vi "GetRow.vi"(0 "reference in":refnum<class "DataGridView.lvclass">, 5 "index":i32, 11 "error in (no error)":errorcluster) -> (4 "reference out":refnum<class "DataGridView.lvclass">, 6 "Array":refnum<k24>[](array[refnum]), 15 "error out":errorcluster)   [LabVIEW 2018, in "DataGridView.lvclass"]
doc: "Gets the row by index"
uses:
  DataGridView.lvclass
  System.Windows.Forms
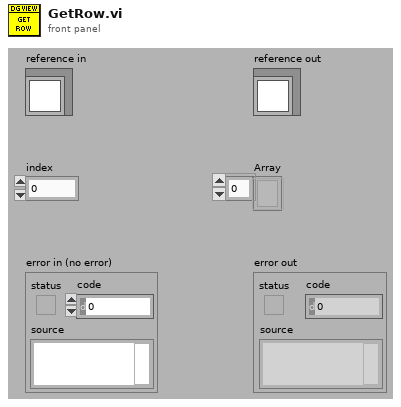
[diagram p1: front panel]
types:
  T1 = typedef "DataGridView.lvclass/ObjectAttributes.ctl" = cluster{"DataGridView":refnum<k24>, "SelectionChangedEvent":refnum<user-event>, "SelectionChanged callback ref":refnum<k27>, "LastSelectedRowIndex":i32}
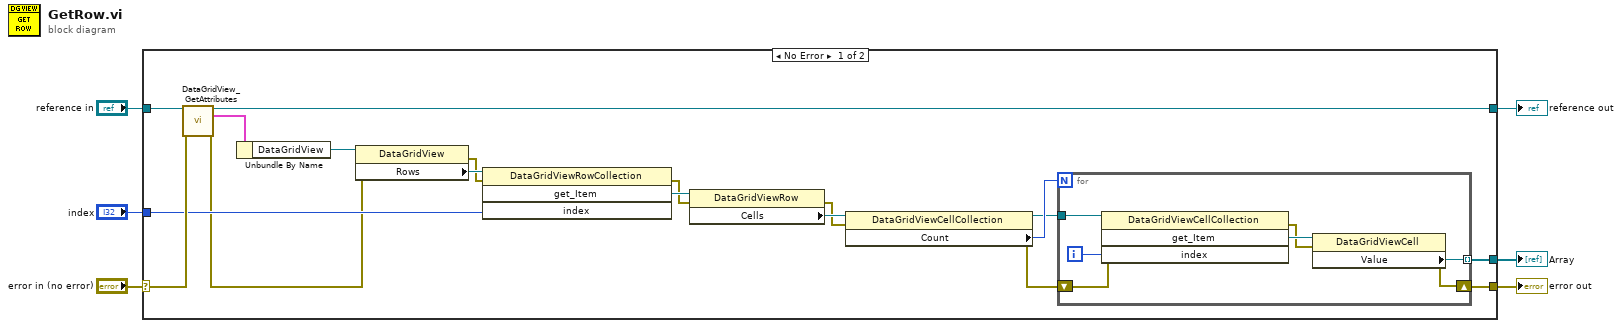
[diagram p0: block diagram]
diagram:
  n1 = case shown="No Error" "error in (no error)" {
    selector: "error in (no error)" -> [w24 w33]
    tunnel: [w12 w33] -> w5
    tunnel: [w21 w32] -> w3
    tunnel: "reference in" -> [w22 w32]
    tunnel: "index" -> [w18 _]
    tunnel: [w13 _] -> w1
    frame No Error {
      n2 = call "DataGridView_GetAttributes.vi"("reference in"=w22, "error in (no error)"=w24) -> ("reference out"=w21:refnum<class "DataGridView.lvclass">, "Data"=w23:T1, "error out"=w11:errorcluster)  [unwired: 10 in, 1 out]
      n3 = Unbundle By Name(w23) -> ("DataGridView"=w20:refnum<k24>)
      n4 = property class="DataGridView"(reference=w20, error in=w11) -> (error out=w8:errorcluster, "Rows"=w19:refnum<k24>)  [unwired: 1 out]
      n5 = invoke class="DataGridViewRowCollection" method="get_Item"(reference=w19, error in=w8, "index"=w18) -> (error out=w9:errorcluster, "get_Item"=w17:refnum<k24>)  [unwired: 1 in, 2 out]
      n6 = property class="DataGridViewRow"(reference=w17, error in=w9) -> (error out=w10:errorcluster, "Cells"=w16:refnum<k24>)  [unwired: 1 out]
      n7 = property class="DataGridViewCellCollection"(reference=w16, error in=w10) -> (reference out=w14:refnum<k24>, error out=w7:errorcluster, "Count"=w15:i32)
      n8 = for {
        N: w15 -> [_]
        tunnel: w14 -> [w31]
        tunnel: [w28] -> w13 mode=indexing
        shift-right: [w25] -> w12
        shift-left: w7 -> [w27]
        i -> [w30]
        n9 = invoke class="DataGridViewCellCollection" method="get_Item"(reference=w31, error in=w27, "index"=w30) -> (error out=w26:errorcluster, "get_Item"=w29:refnum<k24>)  [unwired: 1 in, 2 out]
        n10 = property class="DataGridViewCell"(reference=w29, error in=w26) -> (error out=w25:errorcluster, "Value"=w28:refnum<k24>)  [unwired: 1 out]
      }
    }
    frame Error {
    }
  }
  "error out" <- w5
  "reference out" <- w3
  "Array" <- w1
